vi "CSV Formatter.vi"(8 "error in (no error)":errorcluster, 11 "Byte Stream File in":refnum<file>) -> (0 "error out":errorcluster, 3 "path":path)   [LabVIEW 2016]
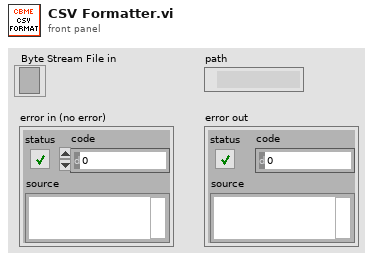
[diagram p1: front panel]
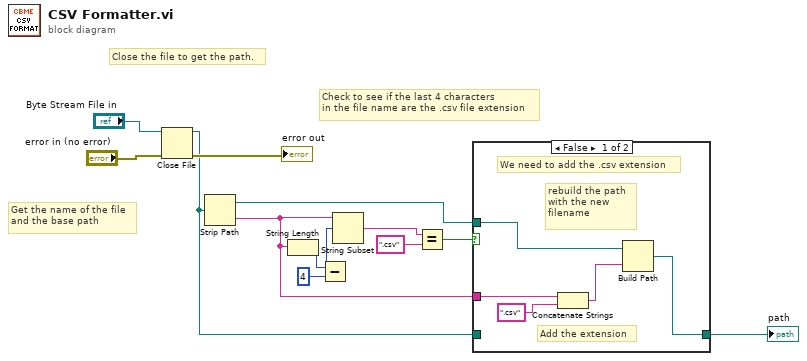
[diagram p0: block diagram]
diagram:
  # "Check to see if the last 4 characters\nin the file name are the .csv file extension"
  # "Get the name of the file\nand the base path"
  # "Close the file to get the path."
  n1 = Close File(refnum="Byte Stream File in", error in="error in (no error)") -> (path=w4:path, error out=→"error out":errorcluster)
  n2 = Strip Path(path=w4) -> (stripped path=w2:path, name=w1:string)
  n3 = String Length(string=w1) -> (length=w11:i32)
  n4 = Subtract(x=w11, y=4) -> (x-y=w13:i32)
  n5 = String Subset(string=w1, offset (0)=w13) -> (substring=w7:string)  [unwired: 1 in]
  n6 = Equal?(x=w7, y=".csv") -> (x = y?=w5:bool)
  n7 = case shown="False" w5 {
    tunnel: w4 -> [_ w19]
    tunnel: [w14 w19] -> w3
    tunnel: w2 -> [w18 _]
    tunnel: w1 -> [w17 _]
    frame False {
      # "rebuild the path \nwith the new \nfilename"
      # "Add the extension"
      # "We need to add the .csv extension"
      n8 = Concatenate Strings(w17, ".csv" ("y")) -> (w15:string)
      n9 = Build Path(base path=w18, name or relative path=w15) -> (appended path=w14:path)
    }
    frame True {
      # "File extension correct\nalready, so pass original\npath through"
    }
  }
  "path" <- w3
